vi "Dequeue.vi"(6 "QueueArrayEntry (QMH)":T2, 7 "DeQueue Type (DeQueue)":T1, 8 "error in (no error)":errorcluster, 10 "timeout in ms (100)":i32=50, 11 "ModuleAdmin In":refnum<class "ModuleAdmin.lvclass">) -> (0 "error out":errorcluster, 1 "timed out?":bool, 2 "Element":variant, 3 "ModuleAdmin Out":refnum<class "ModuleAdmin.lvclass">)   [LabVIEW 2018, in "ModuleAdmin.lvlib" / "ModuleAdmin.lvclass"]
doc: "Dequeues an element from the queue."
uses:
  ModuleAdmin.lvclass
  TypeDefinitions/QueueEntry.ctl
  TypeDefinitions/DeQueueType.ctl
  ModuleAdmin.lvclass/ModuleAdmin.ctl
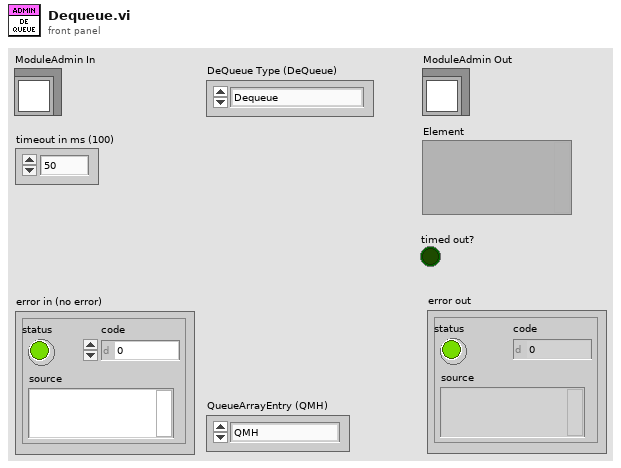
[diagram p1: front panel]
types:
  T1 = typedef "ModuleAdmin.lvlib/ModuleAdmin.lvclass/DeQueueType.ctl" = enum16{"Dequeue", "PreviewQueue"}
  T2 = typedef "ModuleAdmin.lvlib/ModuleAdmin.lvclass/QueueEntry.ctl" = enum16{"QMH", "Class Data", "Data Loop", "Queue 4", "Queue 5", "Queue 6", "Queue 7", "Queue 8", "Queue 9", "Queue 10"}
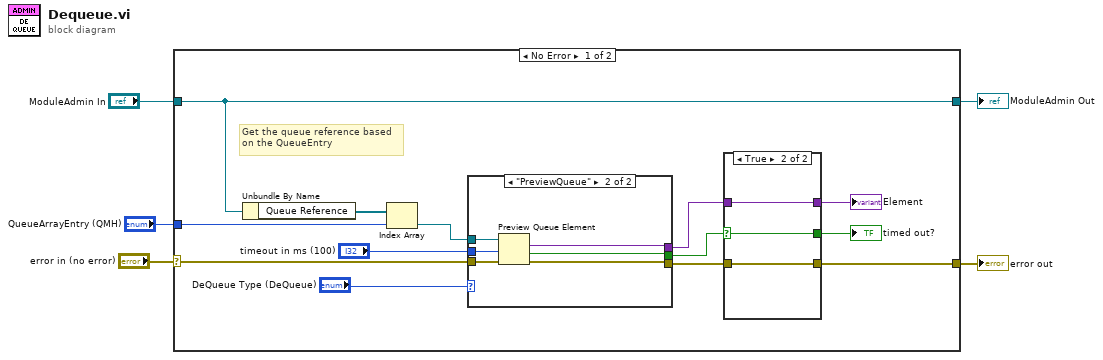
[diagram p0: block diagram]
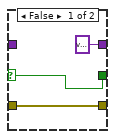
[diagram p2: hidden frame]
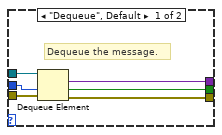
[diagram p3: hidden frame]
diagram:
  n1 = case shown="No Error" "error in (no error)" {
    selector: "error in (no error)" -> [w17 w38]
    tunnel: [w11 w38] -> w5
    tunnel: "QueueArrayEntry (QMH)" -> [w9 _]
    tunnel: "ModuleAdmin In" -> [w8 w37]
    tunnel: [w8 w37] -> w1
    frame No Error {
      # "Get the queue reference based\non the QueueEntry"
      n2 = Unbundle By Name(w8) -> ("Queue Reference"=w7:refnum<queue>[])
      n3 = Index Array(array=w7, index=w9) -> (element=w16:refnum<queue>)
      n4 = case shown="\"PreviewQueue\"" "DeQueue Type (DeQueue)" {
        tunnel: [w30 w34] -> w12
        tunnel: w16 -> [w29 w35]
        tunnel: w17 -> [w28 w36]
        tunnel: [w27 w33] -> w13
        tunnel: "timeout in ms (100)" -> [w26 w31]
        tunnel: [w25 w32] -> w15
        frame "Dequeue", Default {
          # "Dequeue the message."
          n5 = Dequeue Element(queue=w29, timeout in ms (-1)=w26, error in (no error)=w28) -> (element=w27:variant, timed out?=w25:bool, error out=w30:errorcluster)  [unwired: 1 out]
        }
        frame "PreviewQueue" {
          n6 = Preview Queue Element(queue=w35, timeout in ms (-1)=w31, error in (no error)=w36) -> (element=w33:variant, timed out?=w32:bool, error out=w34:errorcluster)  [unwired: 1 out]
        }
      }
      n7 = case shown="True" w15 {
        selector: w15 -> [w21 w24]
        tunnel: [w21 w24] -> w14
        tunnel: w13 -> [_ w22]
        tunnel: w12 -> [w20 w23]
        tunnel: [w20 w23] -> w11
        tunnel: [variant ("element data type") w22] -> w10
        frame False {
        }
        frame True {
        }
      }
      "timed out?" <- w14
      "Element" <- w10
    }
    frame Error {
    }
  }
  "error out" <- w5
  "ModuleAdmin Out" <- w1
